vi "Process ForwardRight.vi"(8 "error in (no error)":errorcluster, 9 "Right":dbl(slide) scale=-1.0..1.0, 10 "Forward":dbl(slide) scale=-1.0..1.0, 11 "Driver in":refnum<class "Driver.lvclass">) -> (0 "error out":errorcluster, 3 "Driver out":refnum<class "Driver.lvclass">)   [LabVIEW 2013, in "Driver.lvlib" / "Driver.lvclass"]
uses:
  Driver.lvclass
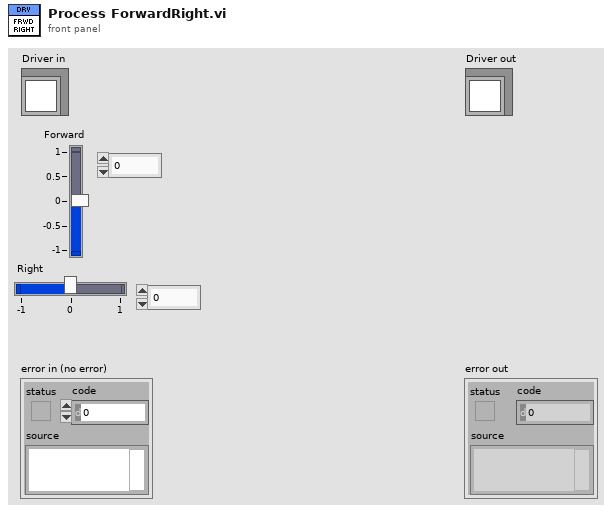
[diagram p1: front panel]
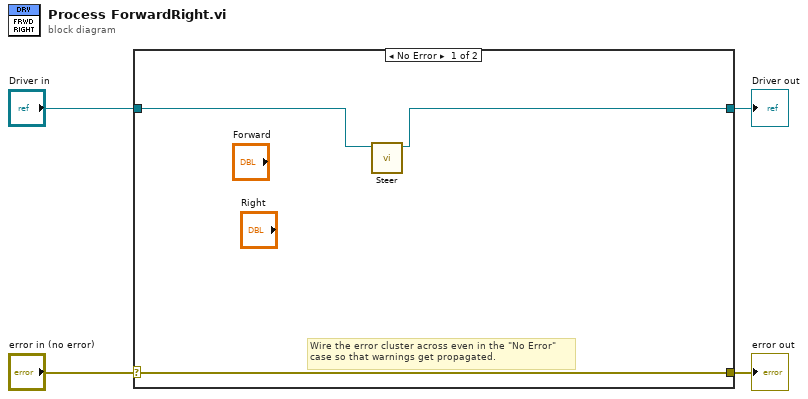
[diagram p0: block diagram]
diagram:
  n1 = case shown="No Error" "error in (no error)" {
    selector: "error in (no error)" -> [w7 w9]
    tunnel: [w7 w9] -> w3
    tunnel: [w5 w8] -> w1
    tunnel: "Driver in" -> [w6 w8]
    frame No Error {
      # "Wire the error cluster across even in the \"No Error\"\ncase so that warnings get propagated."
      n2 = call-dynamic "Steer.vi"("Driver in"=w6) -> ("Driver out"=w5:refnum<class "Driver.lvclass">)  [unwired: 9 in, 1 out]
    }
    frame Error {
    }
  }
  "error out" <- w3
  "Driver out" <- w1
